vi "Add Service.vi"(8 "error in (no error)":errorcluster, 10 "Service":refnum<class "Service.lvclass">, 11 "Server in":refnum<class "Server.lvclass">) -> (0 "error out":errorcluster, 3 "Server out":refnum<class "Server.lvclass">)   [LabVIEW 2020, in "HTTP Server.lvlib" / "Server.lvclass"]
doc: "Adds a Service to the server so it will be available during requests. Only a single instance of a service type can be registered with a server and if a type of service is registered a second time an error will be generated.\n\nAvoid using shared resources in Services when possible as this will lead to contention between parallel requests and significantly reduce request processing performance."
uses:
  Server.lvclass
  Service/Service.lvclass
  Server.lvclass/Server.ctl
  b471059d-eeb9-4dc6-99ed-b3318ca508da.vi
  b471059d-eeb9-4dc6-99ed-b3318ca508da.vi/dd2842a1-4313-49a6-90f2-c24c0bceb404.vi
  Arguments/_Add Argument.vi
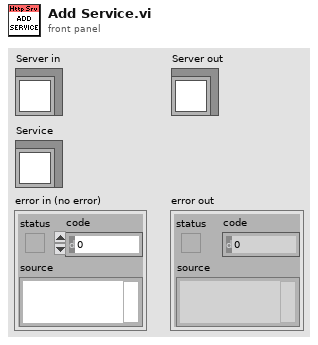
[diagram p1: front panel]
types:
  T1 = typedef "HTTP Server.lvlib/Server.lvclass/Ref Data.ctl" = cluster{"Connection Handler Map":T2, "Request Handler Map":T4, "Route Handler Map":T5, "Controller Handler Map":T6, "Controller Map":T7, "Response Handler Map":T8, "Complete Handler Map":T9, "Exception Handler Map":T10, "Connection Handler Index":u16, "Request Handler Index":u16, "Route Handler Index":u16, "Controller Handler Index":u16, "Controller Index":u16, "Response Handler Index":u16, "Complete Handler Index":u16, "Exception Handler Index":u16, "Services":refnum<class "Arguments.lvclass">, "Path":path, "Session Type":refnum<class "Session.lvclass">, "Session Cookie Name":string, "WebSocket Handler":refnum<class "WebSocket Handler.lvclass">, "WebSocket Handling":bool}
  T2 = typedef "HTTP Server.lvlib/Connection Handler Map.ctl" = map{T3, refnum<class "Connection Handler.lvclass">}
  T3 = typedef "HTTP Server.lvlib/Priority.ctl" = cluster{"Entity":u16, "Index":u16}
  T4 = typedef "HTTP Server.lvlib/Request Handler Map.ctl" = map{T3, refnum<class "Request Handler.lvclass">}
  T5 = typedef "HTTP Server.lvlib/Route Handler Map.ctl" = map{T3, refnum<class "Route Handler.lvclass">}
  T6 = typedef "HTTP Server.lvlib/Controller Handler Map.ctl" = map{T3, refnum<class "Controller Handler.lvclass">}
  T7 = typedef "HTTP Server.lvlib/Controller Map.ctl" = map{T3, refnum<class "Controller.lvclass">}
  T8 = typedef "HTTP Server.lvlib/Response Handler Map.ctl" = map{T3, refnum<class "Response Handler.lvclass">}
  T9 = typedef "HTTP Server.lvlib/Complete Handler Map.ctl" = map{T3, refnum<class "Complete Handler.lvclass">}
  T10 = typedef "HTTP Server.lvlib/Exception Handler Map.ctl" = map{T3, refnum<class "Exception Handler.lvclass">}
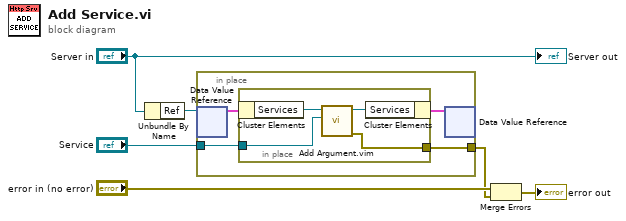
[diagram p0: block diagram]
diagram:
  n1 = Unbundle By Name("Server in") -> ("Ref"=w5:refnum<data-value>)
  n2 = in-place {
    in-place-border: "Service" -> [w8]
    in-place-border: [w7] -> w1
    n3 = in-place-dvr #1(w5) -> (w10:T1)  [unwired: 1 out]
    n4 = in-place {
      in-place-border: w8 -> [w11]
      in-place-border: [w12] -> w7
      n5 = in-place-cluster #2(w10) -> ("Services"=w14:refnum<class "Arguments.lvclass">)
      n6 = call "Add Argument.vim"("Name / Service / Object"=w11, "Arguments in"=w14) -> ("error out"=w12:errorcluster, "Arguments out"=w13:refnum<class "Arguments.lvclass">)  [unwired: 8 in]
      n7 = in-place-cluster #2("Services"=w13) -> (w9:T1)
    }
    n8 = in-place-dvr #1(w9) -> ()  [unwired: 2 out]
  }
  n9 = Merge Errors("error in (no error)", w1) -> (→"error out":errorcluster)
  "Server out" <- "Server in"
